vi "簇转换为字符串数组 (子VI).vi"(11 "簇":T1) -> (3 "数组":string[](array[string]))   [LabVIEW 2016]
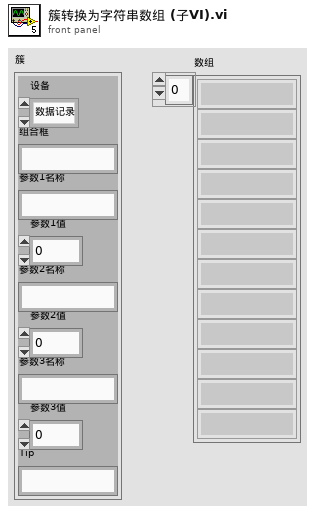
[diagram p1: front panel]
types:
  T1 = cluster{"设备":enum16{"数据记录", "Module", "VICI Valve", "其他"}, "组合框":string, "参数1名称":string, "参数1值":dbl, "参数2名称":string, "参数2值 ":dbl, "参数3名称 ":string, "参数3值  ":dbl, "Tip":string}
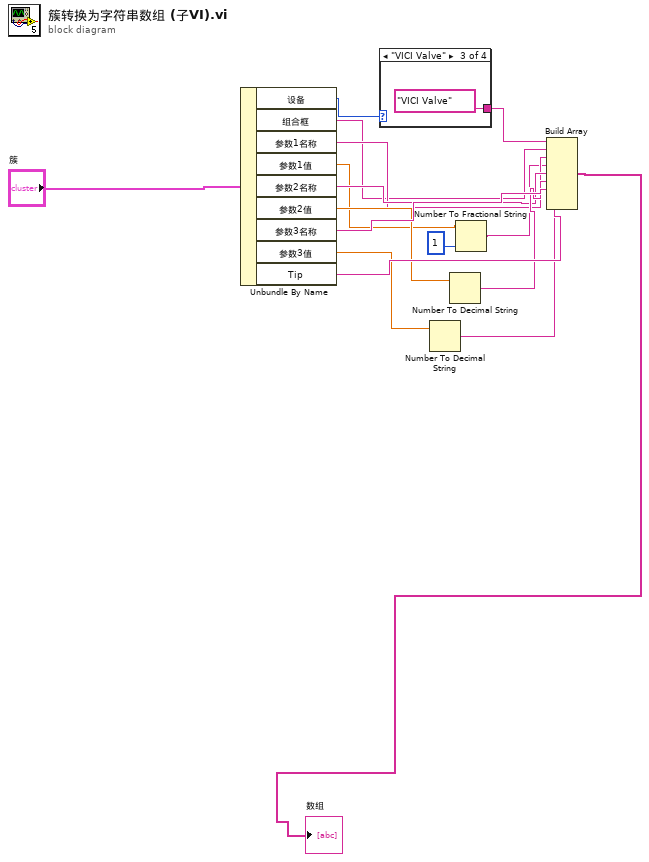
[diagram p0: block diagram]
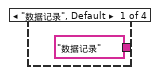
[diagram p2: hidden frame]
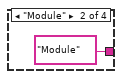
[diagram p3: hidden frame]
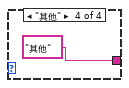
[diagram p4: hidden frame]
diagram:
  n1 = Unbundle By Name("簇") -> ("设备"=w4:enum16{"数据记录", "Module", "VICI Valve", "其他"}, "组合框"=w6:string, "参数1名称"=w7:string, "参数1值"=w3:dbl, "参数2名称"=w8:string, "参数2值"=w9:dbl, "参数3名称"=w11:string, "参数3值"=w12:dbl, "Tip"=w14:string)
  n2 = case shown="\"VICI Valve\"" w4 {
    tunnel: ["数据记录" "Module" "VICI Valve" "其他"] -> w5
    frame "数据记录", Default {
    }
    frame "Module" {
    }
    frame "VICI Valve" {
    }
    frame "其他" {
    }
  }
  n3 = Number To Decimal String(number=w12) -> (decimal integer string=w13:string)  [unwired: 1 in]
  n4 = Number To Decimal String(number=w9) -> (decimal integer string=w10:string)  [unwired: 1 in]
  n5 = Number To Fractional String(number=w3, precision (6)=i16 1 ("宽度(-)")) -> (F-format string=w2:string)  [unwired: 2 in]
  n6 = Build Array(w5, w6, w7, w2, w8, w10, w11, w13, w14) -> (→"数组":string[])
